vi "test.vi"() -> ()   [LabVIEW 2018]
uses:
  Channel Pub/Channel Pub.lvclass
  C:/Users/Denis/Desktop/communication-manager/communication-manager/Communication Channel/Communication Channel Folder/Communication Channel.lvclass
  <vilib>/addons/zeromq/zmq_context.lvclass
  Communication Channel/Communication Channel Folder/Communication Channel.lvclass
panel:
  out "error out":errorcluster
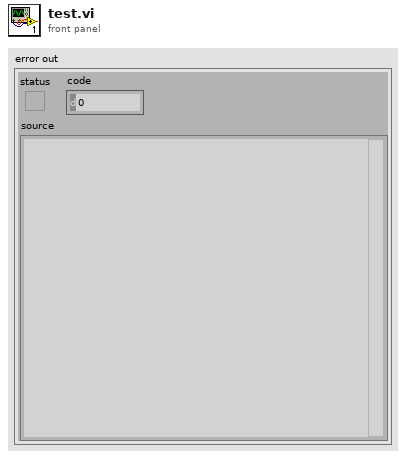
[diagram p1: front panel]
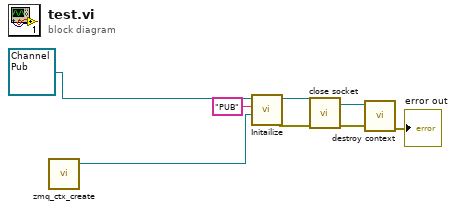
[diagram p0: block diagram]
diagram:
  n1 = call <vilib>:"zmq_ctx_create.vi"() -> ("context out"=w6:refnum<class "zmq_context.lvclass">)  [unwired: 4 in, 1 out]
  n2 = call-dynamic "Initailize.vi"("zeromq.lvlib:ZeroMQ Context"=w6, "Name"="PUB", "Channel Pub in"=refnum<class "Channel Pub.lvclass"> refnum ("Channel Pub.lvclass")) -> ("error out"=w4:errorcluster, "Channel Pub out"=w5:refnum<class "Channel Pub.lvclass">)  [unwired: 7 in]
  n3 = call "close socket.vi"("error in (no error)"=w4, "Communication Channel in"=w5) -> ("error out"=w3:errorcluster, "Communication Channel out"=w2:refnum<class "Channel Pub.lvclass">)  [unwired: 8 in]
  n4 = call "destroy context.vi"("error in (no error)"=w3, "Communication Channel in"=w2) -> ("error out"=→"error out":errorcluster)  [unwired: 8 in, 1 out]
